vi "NanotecSMCPD.set axis position.vi"(0 "i ref in":refnum<vi>, 1 "axis":i32, 2 "position":dbl=1.0, 3 "ms timeout (10000)":i32=10000, 5 "error in (no error)":errorcluster) -> (14 "i ref out":refnum<vi>, 17 "timed out":bool, 19 "error out":errorcluster)   [LabVIEW 2014, in "NanotecSMCPD.lvlib"]
doc: "Sets the value of the position counter of the specified axis. This method does not move the axis. Comment: One can only set the position counter to 0."
uses:
  NanotecSMCPD.lvlib
  CSCore/CSSystem/CoreDefs/CoreDefs.error_type.ctl
  CSCore/CSSystem/CoreDefs/CoreDefs.error_severity.ctl
  CSCore/CSApplicationBaseClasses/MotorBase/MotorBase.directionType.ctl
  CSCore/CSApplicationBaseClasses/MotorBase/MotorBase.serviceType.ctl
  CSCore/CSApplicationBaseClasses/MotorBase/MotorBase.statusType.ctl
  CSlibraries/UtilityLib/UtilityLib.valueStatus.ctl
  CSCore/CSApplicationBaseClasses/DeviceBase/DeviceBase.lvlib
  CSCore/CSSystem/CoreLib/CoreLib.lvlib
  CSCore/CSApplicationBaseClasses/MotorBase/MotorBase.lvlib
  CSlibraries/UtilityLib/UtilityLib.lvlib
  CSinstr.lib/NanotecSMCPD/NanotecSMCPDDriver.lvlib
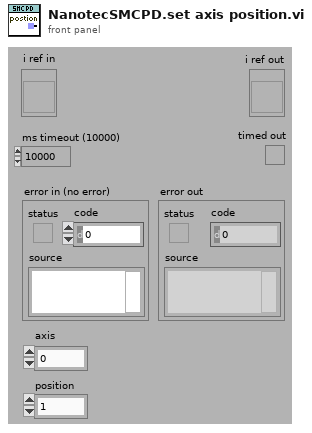
[diagram p1: front panel]
types:
  T1 = typedef "CoreDefs.error_severity.ctl" = enum16{"undefined", "information", "warning", "error", "fatal"}
  T2 = typedef "CoreDefs.error_type.ctl" = enum16{"no error", "can't load process", "can't unload process", "process does not exist", "can't install process", "can't remove process", "unknown function", "time out", "can't execute function", "duplicate queue name", "super not found", "caller queue invalid", "can't ping process", "unknown error", "VISA Error", "VISA timeout", "GPIB timeout", "GPIB error", "communication error", "data type mismatch", "can't read data from OPC server", "can't write data to OPC server", "OET error", "function not implemented", "process already exists", "invalid Shared Variable name", "error writing Shared Variable", "error reading Shared Variable", "invalid client name", "corrupt database", "unknown class", "call not authorized", "parameter out of range", "OET timeout: can't get data to modify", "invalid queue name", "requested operation incompatible with current state", "event undefined", "event disabled", "state undefined", "caller is not a friend", "EventBuilder: bad eventID", "EventBuilder: no DAQ devices", "a thread must not stop itself", "UNUSED ELEMENT4", "DiscArchiver: eventData incomplete", "DiscArchiver: eventData does not belong to run", "DiscArchiver: can't open file", "DiscArchiver: can't write to file", "DiscArchiver: available disc space low", "can't acquire semaphore", "error reading data from database", "notifier object is not existing", "can't register process", "can't unregister process", "illegal event type", "object disabled", "object already exists", "can't change state", "Instrument not found", "no connection to remote node", "invalid reference", "N/A", "UNUSED ELEMENT 1", "element not found", "illegal TCP/IP connection detected", "object does not exist", "invalid access ID", "unknown CS system", "invalid privilige", "unsupported data type", "unsupported server type", "IO server already exists", "Shared Variable already exists"}
  T3 = typedef "UtilityLib.lvlib/UtilityLib.valueStatus.ctl" = enum16{"no info available", "stand by/off", "on", "warning", "alarm/malfunction", "not implemented", "user action required", "important information", "system default", "control default", "indicator default", "button default"}
  T4 = typedef "MotorBase.lvlib/MotorBase.serviceType.ctl" = enum16{"onOff", "startVelocity", "stopVelocity", "acceleration", "rangeMin", "rangeMax", "status", "position"}
  T5 = typedef "MotorBase.lvlib/MotorBase.directionType.ctl" = enum16{"unknown", "update actual value", "update nominal value", "update both"}
  T6 = typedef "MotorBase.lvlib/MotorBase.statusType.ctl" = u32
  T7 = typedef "MotorBase.lvlib/MotorBase.i attribute.ctl" = cluster{"defaultAxisIndex":i32, "logicalName":string[], "nOfAxes":i32, "physicalName":string[], "scaling":dbl[], "units":string[], "defaulAxisIndexID":i32, "logicalNameID":i32, "nOfAxesID":i32, "physicalNameID":i32, "unitID":i32, "actValues":T8, "nomValues":T8}
  T8 = typedef "MotorBase.lvlib/MotorBase.parameters.ctl" = cluster{"services":cluster{"onOff":bool[], "startVelocity":dbl[], "stopVelocity":dbl[], "acceleration":dbl[], "rangeMin":dbl[], "rangeMax":dbl[], "status":T6[], "position":dbl[]}, "serviceIDs":cluster{"onOffID":i32, "startVelocityID":i32, "stopVelocityID":i32, "accelerationID":i32, "rangeMinID":i32, "rangeMaxID":i32, "statusID":i32, "positionID":i32}}
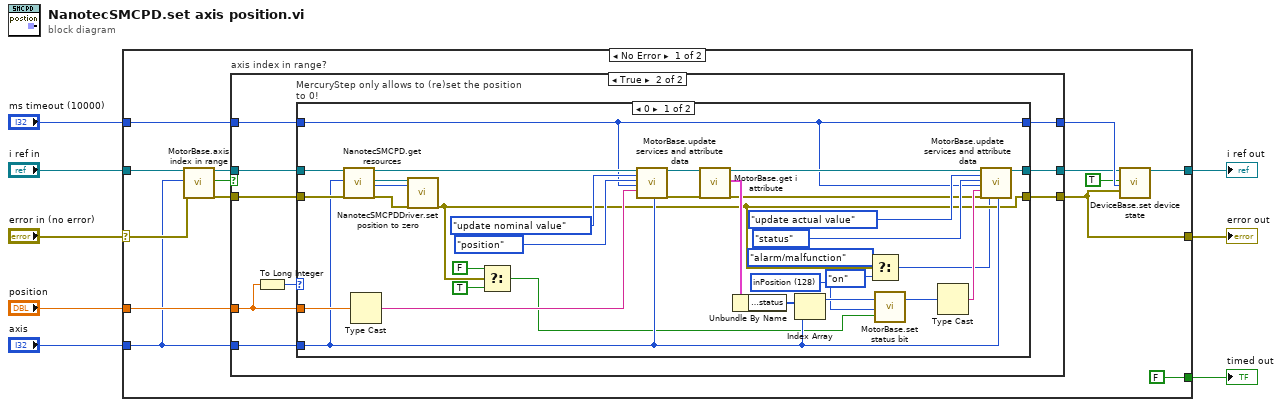
[diagram p0: block diagram]
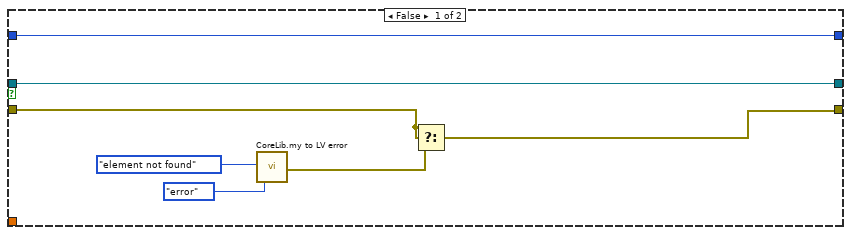
[diagram p2: hidden frame]
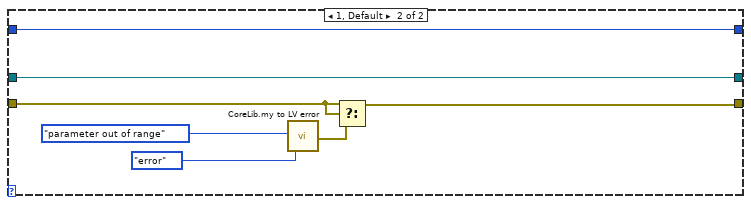
[diagram p3: hidden frame]
diagram:
  n1 = case shown="No Error" "error in (no error)" {
    selector: "error in (no error)" -> [w15 w78]
    tunnel: "ms timeout (10000)" -> [w11 _]
    tunnel: "i ref in" -> [w16 w79]
    tunnel: [w14 w78] -> w5
    tunnel: "axis" -> [w12 _]
    tunnel: [w10 w79] -> w3
    tunnel: "position" -> [w13 _]
    tunnel: [FALSE ("timed out") _] -> w1
    frame No Error {
      n2 = call "MotorBase.axis index in range.vi"("i ref in"=w16, "axisIndex"=w12, "error in (no error)"=w15) -> ("i ref out"=w20:refnum<vi>, "in range"=w19:bool, "error out"=w21:errorcluster)  [unwired: 14 in]
      n3 = case "axis index in range?" shown="True" w19 {
        tunnel: [w29 w35] -> w18
        tunnel: [w26 w34] -> w14
        tunnel: w11 -> [w23 w36]
        tunnel: w13 -> [_ w31]
        tunnel: w12 -> [_ w33]
        tunnel: w20 -> [w29 w38]
        tunnel: w21 -> [w27 w37]
        tunnel: [w23 w30] -> w22
        frame False {
          n4 = call "CoreLib.my to LV error.vi"("ErrorTypes"=CoreDefs.error_type."element not found", "severityLevel"=CoreDefs.error_severity."error") -> ("myErrorCluster"=w25:errorcluster)  [unwired: 16 in, 1 out]
          n5 = Select(t=w27, s=w27, f=w25) -> (s? t:f=w26:errorcluster)
        }
        frame True {
          n6 = To Long Integer(number=w31) -> (32bit integer=w32:i32)
          n7 = case "MercuryStep only allows to (re)set the position to 0!" shown="0" w32 {
            tunnel: w38 -> [w56 w72]
            tunnel: w37 -> [w55 w77]
            tunnel: w36 -> [w47 w71]
            tunnel: [w68 w72] -> w35
            tunnel: [w43 w73] -> w34
            tunnel: w33 -> [w54 _]
            tunnel: w31 -> [w57 _]
            tunnel: [w47 w71] -> w30
            frame 0 {
              w48 = T6 128 items=["motorEnabled"=1, "negativeLimitSwitchActive"=2, "positiveLimitSwitchActive"=4, "limitSwitchesEnabled"=8, "limitSwitchesAreNormallyClosed"=16, "reseved1"=32, "referenced"=64, "inPosition"=128, "reserved2"=256, "reserved3"=512, "reserved4"=1024, "reserved5"=2048, "error"=4096, "reserved6"=8192, "reserved7"=16384, "reserved8"=32768, "user defined1"=65536, "user defined2"=131072, "user defined3"=262144, "user defined4"=524288, "user defined5"=1048576, "user defined6"=2097152, "user defined7"=4194304, "user defined8"=8388608, "user defined9"=16777216, "user defined10"=33554432, "user defined11"=67108864, "user defined12"=134217728, "user defined13"=268435456, "user defined14"=536870912, "user defined15"=1073741824, "user defined16"=2147483648] ("service")
              n8 = call "NanotecSMCPD.get resources.vi"("i ref in"=w56, "axisNumber"=w54, "error in (no error)"=w55) -> ("i ref out"=w51:refnum<vi>, "VISA resource"=w53:refnum<visa-resource-name>, "address"=w39:i32, "error out"=w52:errorcluster)  [unwired: 13 in]
              n9 = Type Cast(x=w57) -> (*(type *) &x=w70:string)  [unwired: 1 in]
              n10 = call "NanotecSMCPDDriver.set position to zero.vi"("VISA resource name"=w53, "contollerID"=w39, "error in (no error)"=w52) -> ("error out"=w43:errorcluster)  [unwired: 14 in, 2 out]
              n11 = Select(t=FALSE, s=w43, f=TRUE ("setBit")) -> (s? t:f=w44:bool)
              n12 = call "MotorBase.update services and attribute data.vi"("i ref in"=w51, "direction"=MotorBase.directionType."update nominal value", "service"=MotorBase.serviceType."position", "ms timeout (10000)"=w47, "value"=w70, "axisNumber"=w54) -> ("i ref out"=w65:refnum<vi>, "error out"=w64:errorcluster)  [unwired: 11 in, 1 out]
              n13 = call "MotorBase.get i attribute.vi"("i ref in"=w65, "error in (no error)"=w64) -> ("i ref out"=w61:refnum<vi>, "i attribute"=w63:T7, "error out"=w60:errorcluster)  [unwired: 15 in]
              n14 = Unbundle By Name(w63) -> ("actValues.services.status"=w62:T6[])
              n15 = Index Array(array=w62, index=w54) -> (element=w49:T6)
              n16 = Select(t=UtilityLib.valueStatus."alarm/malfunction", s=w43, f=UtilityLib.valueStatus."on" ("quality")) -> (s? t:f=w40:T3)
              n17 = call "MotorBase.set status bit.vi"("status"=w49, "statusBit"=w48, "setBit"=w44) -> ("status out"=w50:T6)  [unwired: 16 in]
              n18 = Type Cast(x=w50) -> (*(type *) &x=w69:string)  [unwired: 1 in]
              n19 = call "MotorBase.update services and attribute data.vi"("i ref in"=w61, "direction"=MotorBase.directionType."update actual value", "service"=MotorBase.serviceType."status", "ms timeout (10000)"=w47, "value"=w69, "error in (no error)"=w60, "quality"=w40, "axisNumber"=w54) -> ("i ref out"=w68:refnum<vi>)  [unwired: 9 in, 2 out]
            }
            frame 1, Default {
              n20 = call "CoreLib.my to LV error.vi"("ErrorTypes"=CoreDefs.error_type."parameter out of range", "severityLevel"=CoreDefs.error_severity."error") -> ("myErrorCluster"=w76:errorcluster)  [unwired: 16 in, 1 out]
              n21 = Select(t=w77, s=w77, f=w76) -> (s? t:f=w73:errorcluster)
            }
          }
        }
      }
      n22 = call "DeviceBase.set device state.vi"("i ref in"=w18, "implicit"=TRUE, "ms timeout (10000)"=w22, "device error"=w14) -> ("i ref out"=w10:refnum<vi>)  [unwired: 13 in, 2 out]
    }
    frame Error {
    }
  }
  "error out" <- w5
  "i ref out" <- w3
  "timed out" <- w1
